vi "Open with Default Program.vi"(8 "error in (no error)":errorcluster, 11 "File Path":path) -> (0 "error out":errorcluster)   [LabVIEW 2024]
doc: "Opens a file with the default program in the operating system."
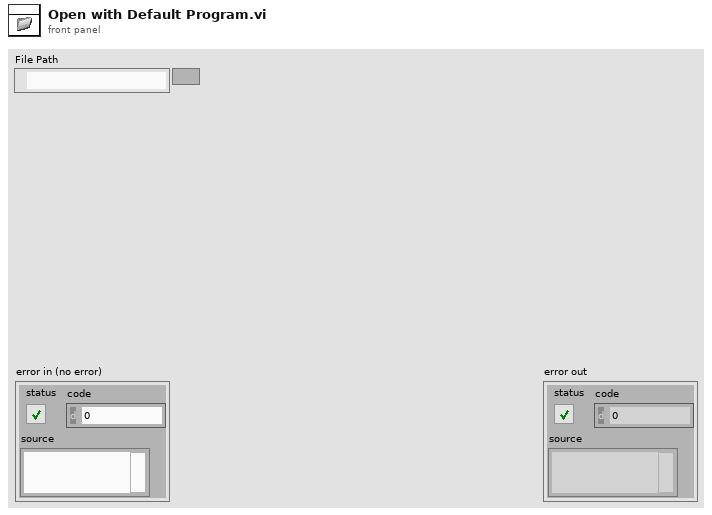
[diagram p1: front panel]
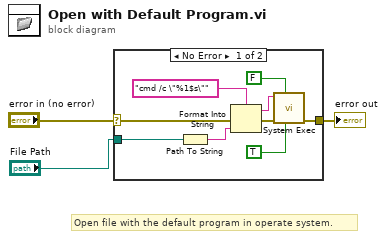
[diagram p0: block diagram]
diagram:
  # "Open file with the default program in operate system."
  n1 = case shown="No Error" "error in (no error)" {
    selector: "error in (no error)" -> [w10 w13]
    tunnel: [w12 w13] -> w2
    tunnel: "File Path" -> [w11 _]
    frame No Error {
      n2 = Path To String(path=w11) -> (string=w7:string)
      n3 = Format Into String(format string="cmd /c \"%1$s\"", error in=w10, w7) -> (resulting string=w5:string, error out=w8:errorcluster)  [unwired: 1 in]
      n4 = call <vilib>:"System Exec.vi"("run minimized? (F)"=TRUE, "wait until completion? (T)"=FALSE, "error in (no error)"=w8, "command line"=w5) -> ("error out"=w12:errorcluster)  [unwired: 4 in, 3 out]
    }
    frame Error {
    }
  }
  "error out" <- w2
